vi "Configure Calibration Outputs.vi"(11 "Controller In":refnum<class "gController.lvclass">) -> ()   [LabVIEW 2018, in "Controller.lvlib" / "gController.lvclass"]
uses:
  gController.lvclass
  C:/Program Files (x86)/National Instruments/LabVIEW 2018/vi.lib/ActorFramework/Actor/Actor.lvclass
  Messages/Update UV Lamp State MSG/Update UV Lamp State MSG.lvclass
  G:/sw_repo/For Builds/Nicholas/Controller/Messages/Generic Boolean MSG/Generic Boolean Message.lvclass
  C:/Program Files (x86)/National Instruments/LabVIEW 2018/vi.lib/ActorFramework/Message/Message.lvclass
  Messages/Update O2 Add MSG/Update O2 Valve State MSG.lvclass
  Messages/Update O3 Valve State MSG/Update O3 Valve State MSG.lvclass
  Messages/Generic Boolean MSG/Generic Boolean Message.lvclass/Generic Boolean Message.ctl
  <vilib>/ActorFramework/Actor/Actor.lvclass/Actor.ctl
  <vilib>/ActorFramework/Message Enqueuer/Message Enqueuer.lvclass/Message Enqueuer.ctl
  Messages/Generic Boolean MSG/Write Bool.vi
  <vilib>/ActorFramework/Message Enqueuer/Init from Existing Queue.vi
  <vilib>/ActorFramework/Message Priority Queue/Priority Enqueue.vi
  <vilib>/ActorFramework/Message Enqueuer/Message Enqueuer.lvclass
  <vilib>/ActorFramework/Actor/Actor.lvclass
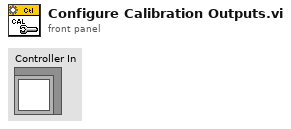
[diagram p1: front panel]
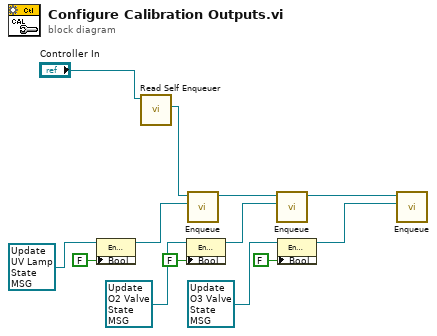
[diagram p0: block diagram]
diagram:
  n1 = property class="Enable UV Lamp MSG"(reference=refnum<class "Update UV Lamp State MSG.lvclass"> refnum ("Controller.lvlib:Enable UV Lamp MSG"), "Bool"=FALSE) -> (reference out=w6:refnum<class "Update UV Lamp State MSG.lvclass">)  [unwired: 1 in, 1 out]
  n2 = call <vilib>:"Read Self Enqueuer.vi"("Actor"="Controller In") -> ("Self Enqueuer"=w1:refnum<class "Message Enqueuer.lvclass">)  [unwired: 10 in]
  n3 = property class="Enable O2 Add Valve MSG"(reference=refnum<class "Update O2 Valve State MSG.lvclass"> refnum ("Controller.lvlib:Enable O2 Add Valve MSG"), "Bool"=FALSE) -> (reference out=w7:refnum<class "Update O2 Valve State MSG.lvclass">)  [unwired: 1 in, 1 out]
  n4 = call <vilib>:"Enqueue.vi"("Message"=w6, "Message Enqueuer in"=w1) -> ("Message Enqueuer out"=w8:refnum<class "Message Enqueuer.lvclass">)  [unwired: 8 in, 1 out]
  n5 = call <vilib>:"Enqueue.vi"("Message"=w7, "Message Enqueuer in"=w8) -> ("Message Enqueuer out"=w10:refnum<class "Message Enqueuer.lvclass">)  [unwired: 8 in, 1 out]
  n6 = property class="Enable Compressor MSG"(reference=refnum<class "Update O3 Valve State MSG.lvclass"> refnum ("Controller.lvlib:Enable Compressor MSG"), "Bool"=FALSE) -> (reference out=w9:refnum<class "Update O3 Valve State MSG.lvclass">)  [unwired: 1 in, 1 out]
  n7 = call <vilib>:"Enqueue.vi"("Message"=w9, "Message Enqueuer in"=w10) -> ()  [unwired: 8 in, 2 out]
